vi "TesteCliente.vi"() -> ()   [LabVIEW 2012]
uses:
  Typedefs/Tipo_PacoteModuloCRIO.ctl
  Typedefs/Tipo_moduloCRIO.ctl
  <vilib>/NI/STM/TCP/Read Meta Data (TCP Ref).vi
  <vilib>/NI/STM/TCP/Read Meta Data (TCP Clst).vi
  <vilib>/NI/STM/TCP/Write Message (TCP).vi
  <vilib>/NI/STM/TCP/Read Message (TCP).vi
  <vilib>/NI/STM/NI STM.lvlib
panel:
  out "value":T1[](array[typedef])
  in  "stop":bool
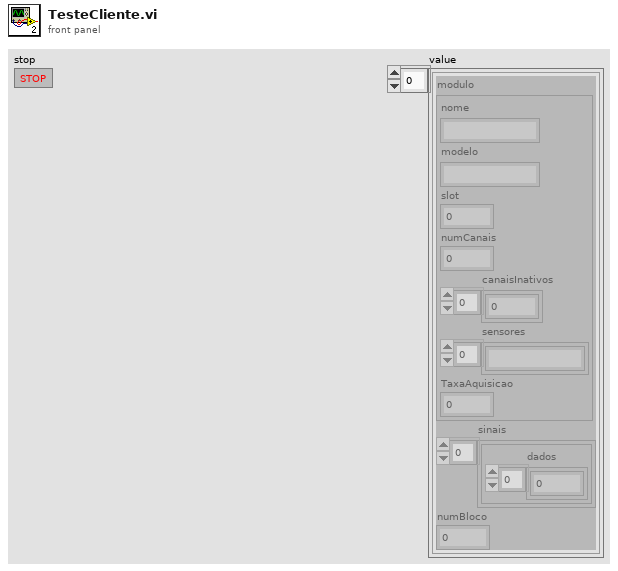
[diagram p1: front panel]
types:
  T1 = typedef "Tipo_PacoteModuloCRIO.ctl" = cluster{"modulo":T2, "sinais":cluster{"dados":sgl[]}[], "numBloco":i32}
  T2 = typedef "Tipo_moduloCRIO.ctl" = cluster{"nome":string, "modelo":string, "slot":i32, "numCanais":i32, "canaisInativos":i32[], "sensores":string[], "TaxaAquisicao":dbl}
  T3 = typedef "NI STM.lvlib/MetaDataElement.ctl" = string
  T4 = typedef "NI STM.lvlib/TCP Connection Info.ctl" = cluster{"connection ID":refnum<k5>, "meta data":T3[]}
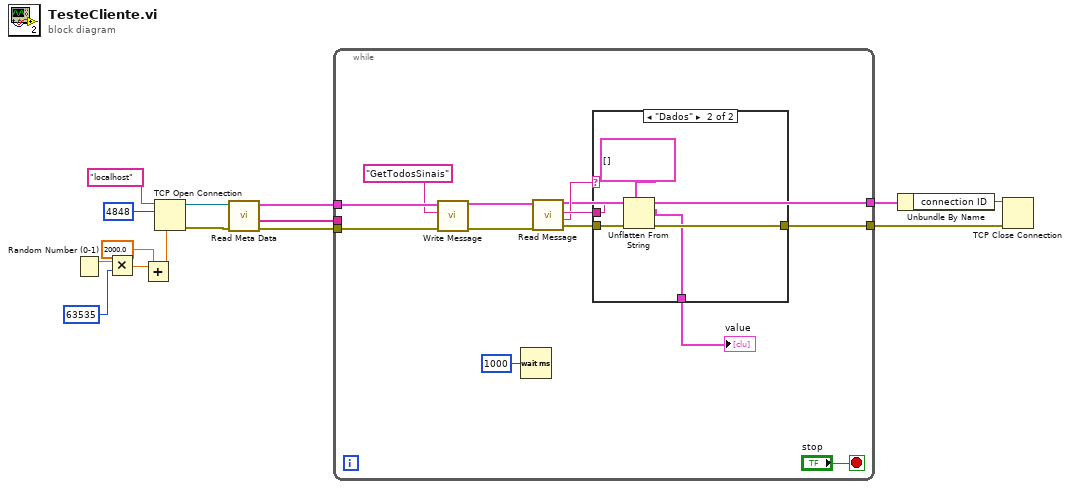
[diagram p0: block diagram]
diagram:
  n1 = Random Number (0-1)() -> (number: 0 to 1=w5:dbl)
  n2 = Multiply(x=w5, y=u16 63535) -> (x*y=w3:dbl)
  n3 = Add(x=w3, y=2000.0) -> (x+y=w1:dbl)
  n4 = TCP Open Connection(address="localhost" ("Target IP Address"), remote port or service name=u16 4848 ("remote port"), local port=w1) -> (connection ID=w13:refnum<k5>, error out=w12:errorcluster)  [unwired: 2 in]
  n5 = call-poly <vilib>:"Read Meta Data.vi"("error in"=w12, "connection ID"=w13) -> ("error out"=w10:errorcluster, "meta data"=w9:T3[], "connection info out"=w11:T4)  [unwired: 7 in]
  n6 = while {
    tunnel: w11 -> [w28]
    tunnel: w10 -> [w27]
    tunnel: w9 -> [_]
    tunnel: [w19] -> w8
    tunnel: [w16] -> w7
    stop <- "stop" stop-if-true
    n7 = call-poly <vilib>:"Write Message.vi"("error in"=w27, "name"="GetTodosSinais", "connection info in"=w28) -> ("error out"=w23:errorcluster, "connection info out"=w24:T4)  [unwired: 7 in]
    n8 = Wait (ms)(milliseconds to wait=u32 1000) -> ()  [unwired: 1 out]
    n9 = call-poly <vilib>:"Read Message.vi"("error in"=w23, "connection info in"=w24) -> ("error out"=w20:errorcluster, "name"=w21:T3, "data string"=w22:string, "connection info out"=w16:T4)  [unwired: 4 in, 2 out]
    n10 = case shown="\"Dados\"" w21 {
      tunnel: w22 -> [_ w34]
      tunnel: w20 -> [w29 w33]
      tunnel: [w29 w32] -> w19
      tunnel: [_ w30] -> w18
      frame Default {
      }
      frame "Dados" {
        n11 = Unflatten From String(type=T1[] [], binary string=w34, error in (no error)=w33) -> (value=w30:T1[], error out=w32:errorcluster)  [unwired: 2 in, 1 out]
      }
    }
    "value" <- w18
  }
  n12 = Unbundle By Name(w7) -> ("connection ID"=w6:refnum<k5>)
  n13 = TCP Close Connection(connection ID=w6, error in (no error)=w8) -> ()  [unwired: 1 in, 2 out]
